vi "Imform Ready Out.vi"(11 "Main Ref":T1) -> (3 "Flow Out":bool)   [LabVIEW 2019, in "MPC_Laser Marked.lvclass"]
uses:
  MPC_Laser Marked.lvclass
  Function/IO Folder/IO_VI/IOCtrl/Ctrl/DMC1000B_1 SelectIn.ctl
  LLB/Commonly VI.lvlib
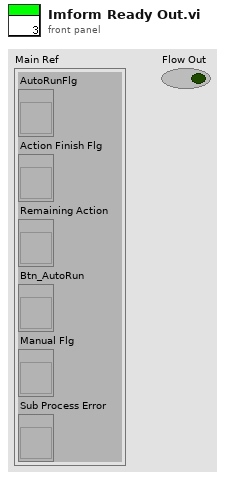
[diagram p1: front panel]
types:
  T1 = cluster{"AutoRunFlg":refnum<vi>, "Action Finish Flg":refnum<vi>, "Remaining Action":refnum<vi>, "Btn_AutoRun":refnum<vi>, "Manual Flg":refnum<vi>, "Sub Process Error":refnum<vi>}
  T2 = typedef "DMC1000B_1 SelectIn.ctl" = enum16{"M_IN00預備", "M_IN01緊急急停檢測", "M_IN02啟動按鈕綠色", "M_IN03正壓氣壓檢知", "M_IN04安全門感知", "M_IN05接受前機台有料#1信號", "M_IN06接受前機台有料#2信號", "M_IN07接受後機台要料#3信號", "M_IN08接受後機台要料#4信號", "M_IN09軌道載板前進料到位檢知", "M_IN10到料阻擋氣缸上位檢知(阻擋位)", "M_IN11到料阻擋氣缸下位檢知(阻擋位)", "M_IN12上頂固定載板氣缸上位檢知", "M_IN13上頂固定載板氣缸下位檢知", "M_IN14軌道載板到位減速檢知", "M_IN15軌道載板到位檢知", "M_IN16軌道載板後出料檢知", "M_IN17", "M_IN18", "M_IN19", "M_IN20", "M_IN21第一軸準備輸入信號 RDY", "M_IN22第二軸準備輸入信號 RDY", "M_IN23第三軸準備輸入信號 RDY", "M_IN24", "M_IN25第一軸ALM+(  伺服警報輸出  )", "M_IN26第二軸ALM+(  伺服警報輸出  )", "M_IN27第三軸ALM+(  伺服警報輸出  )", "M_IN28", "M_IN29第一軸定位完成信號 INP", "M_IN30第二軸定位完成信號 INP", "M_IN31第三軸定位完成信號 INP", "M_IN32"}
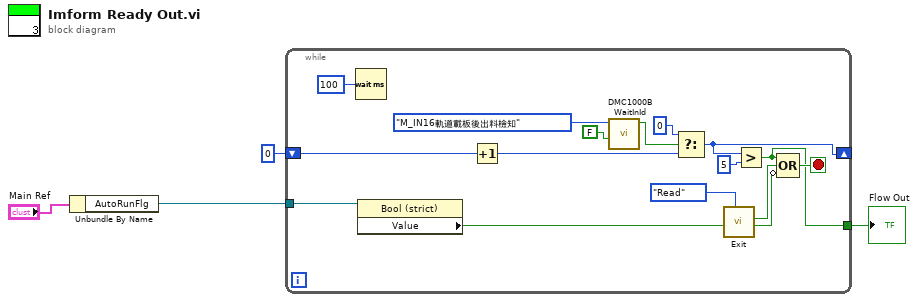
[diagram p0: block diagram]
diagram:
  n1 = Unbundle By Name("Main Ref") -> ("AutoRunFlg"=w4:refnum<vi>)
  n2 = while {
    tunnel: w4 -> [w16]
    shift-right: [w9] -> _
    shift-left: 0 -> [w10]
    tunnel: [w5] -> w1
    stop <- w14 stop-if-true
    n3 = Wait (ms)(milliseconds to wait=u32 100) -> ()  [unwired: 1 out]
    n4 = property class="Bool (strict)"(reference=w16) -> ("Value"=w13:bool)  [unwired: 1 in, 2 out]
    n5 = Increment(x=w10) -> (x+1=w7:i32)
    n6 = call "DMC1000B WaitInId.vi"("Wait?"=FALSE, "64IIN_4 Select"=DMC1000B_1_SelectIn."M_IN16軌道載板後出料檢知") -> ("StatusOut"=w11:bool)  [unwired: 7 in, 2 out]
    n7 = Select(t=0 ("f"), s=w11, f=w7) -> (s? t:f=w9:i32)
    n8 = call "Exit.vi"("Enum"=enum16{"Initial", "Read", "Write"}."Read") -> ("ExitOut"=w15:bool)  [unwired: 10 in]
    n9 = Greater?(x=w9, y=5) -> (0:w5:bool)
    n10 = Compound Arithmetic op=OR(w5, w15, invert w13) -> (w14:bool)
  }
  "Flow Out" <- w1
